vi "GetResolution.vi"(8 "error in (no error)":errorcluster, 11 "CameraTesting in":refnum<class "CameraTesting.lvclass">) -> (0 "error out":errorcluster, 3 "CameraTesting out":refnum<class "CameraTesting.lvclass">)   [LabVIEW 2020, in "CameraTesting.lvlib" / "CameraTesting.lvclass"]
uses:
  CameraTesting.lvclass
  CameraTesting.lvclass/CameraTesting.ctl
  Camera/ICamera/ICamera/ICamera.lvclass
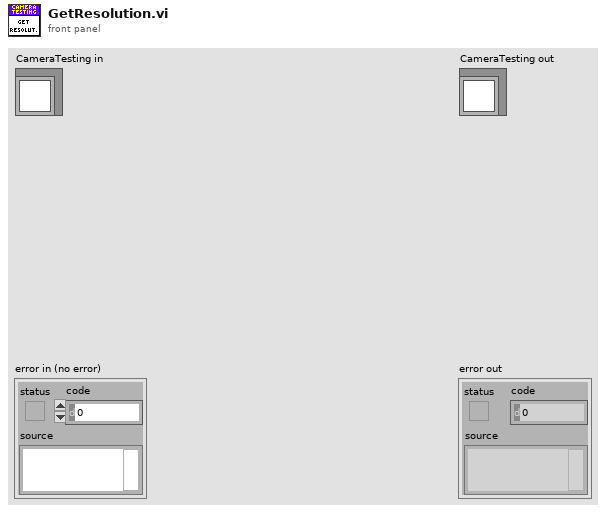
[diagram p1: front panel]
types:
  T1 = typedef "ICameraTesting.lvlib/ICameraTesting.lvclass/ResolutionValReceived.ctl" = refnum<user-event>
  T2 = typedef "ICameraTesting.lvlib/ICameraTesting.lvclass/StatusUpdated.ctl" = refnum<user-event>
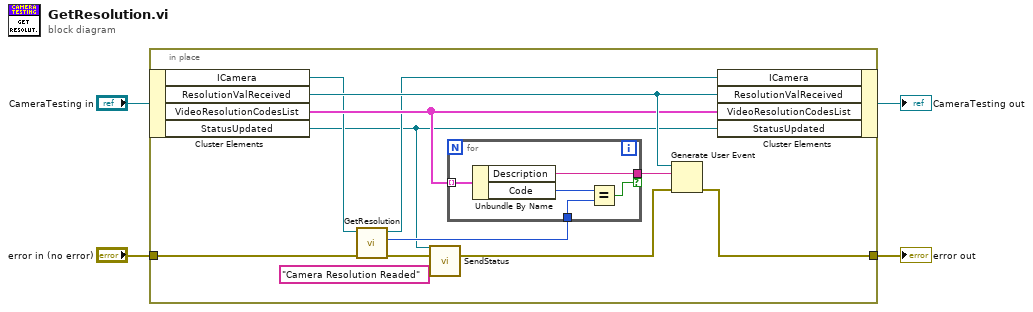
[diagram p0: block diagram]
diagram:
  n1 = in-place {
    in-place-border: "error in (no error)" -> [w11]
    in-place-border: [w15] -> w2
    n2 = in-place-cluster #1("CameraTesting in") -> ("ICamera"=w12:refnum<class "ICamera.lvclass">, "ResolutionValReceived"=w16:T1, "VideoResolutionCodesList"=w14:cluster{"Description":string, "Code":u8}[], "StatusUpdated"=w5:T2)
    n3 = call-dynamic "GetResolution.vi"("error in (no error)"=w11, "ICamera in"=w12) -> ("error out"=w7:errorcluster, "Resolution"=w10:u8, "ICamera out"=w9:refnum<class "ICamera.lvclass">)  [unwired: 7 in]
    n4 = call "SendStatus.vi"("StatusUsrEvn"=w5, "error in"=w7, "Text"="Camera Resolution Readed") -> ("error out"=w6:errorcluster)  [unwired: 24 in]
    n5 = for {
      tunnel: w14 -> [w21] mode=indexing
      tunnel: [w20] -> w13 if=w18
      tunnel: w10 -> [w17]
      n6 = Unbundle By Name(w21) -> ("Description"=w20:string, "Code"=w19:u8)
      n7 = Equal?(x=w19, y=w17) -> (x = y?=w18:bool)
    }
    n8 = Generate User Event(user event=w16, event data cluster=w13, error in=w6) -> (error out=w15:errorcluster)  [unwired: 1 in, 1 out]
    n9 = in-place-cluster #1("ICamera"=w9, "ResolutionValReceived"=w16, "VideoResolutionCodesList"=w14, "StatusUpdated"=w5) -> (→"CameraTesting out":refnum<class "CameraTesting.lvclass">)
  }
  "error out" <- w2
